vi "Set PID Params.vi"(8 "error in (no error)":errorcluster, 9 "Values":dbl[](array[numeric]), 11 "TimedPWMControl in":refnum<class "TimedPWMControl.lvclass">) -> (0 "error out":errorcluster, 3 "TimedPWMControl out":refnum<class "TimedPWMControl.lvclass">)   [LabVIEW 2020, in "VolatusControl.lvlib" / "TimedPWMControl.lvclass"]
uses:
  TimedPWMControl.lvclass
  TimedPWMControl.lvclass/TimedPWMControl.ctl
  lv-control/IG PID/Parameters.ctl
  lv-control/IG PID/IG PID.lvlib
  lv-control/IG PID/PID/PID.lvclass
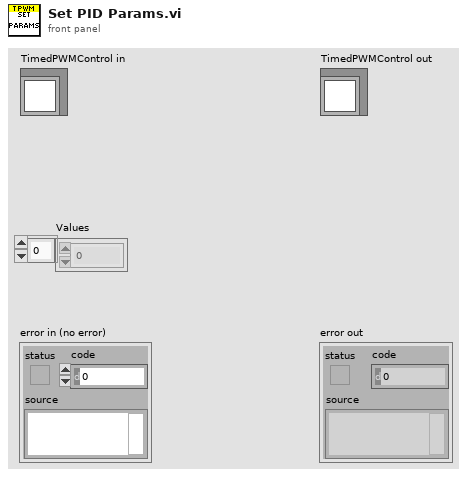
[diagram p1: front panel]
types:
  T1 = typedef "IG PID.lvlib/Parameters.ctl" = cluster{"P Band":dbl, "I Gain":dbl, "D Gain":dbl, "F Gain":dbl}
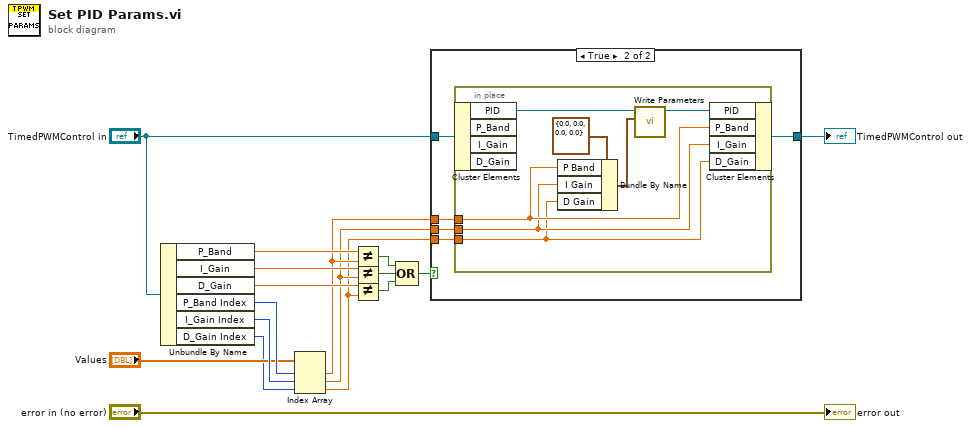
[diagram p0: block diagram]
diagram:
  n1 = Unbundle By Name("TimedPWMControl in") -> ("P_Band"=w13:dbl, "I_Gain"=w14:dbl, "D_Gain"=w12:dbl, "P_Band Index"=w15:i32, "I_Gain Index"=w16:i32, "D_Gain Index"=w2:i32)
  n2 = Index Array(array="Values", index #1=w15, index #2=w16, index #3=w2) -> (element #1=w8:dbl, element #2=w7:dbl, element #3=w3:dbl)
  n3 = Not Equal?(x=w13, y=w8) -> (x != y?=w11:bool)
  n4 = Not Equal?(x=w14, y=w7) -> (x != y?=w10:bool)
  n5 = Not Equal?(x=w12, y=w3) -> (x != y?=w9:bool)
  n6 = Compound Arithmetic op=OR(w11, w10, w9) -> (w1:bool)
  n7 = case shown="True" w1 {
    tunnel: w8 -> [_ w23]
    tunnel: w7 -> [_ w22]
    tunnel: [w18 w21] -> w6
    tunnel: "TimedPWMControl in" -> [w18 w20]
    tunnel: w3 -> [_ w19]
    frame False {
    }
    frame True {
      n8 = in-place {
        in-place-border: w23 -> [w29]
        in-place-border: w22 -> [w28]
        in-place-border: w19 -> [w27]
        n9 = in-place-cluster #1(w20) -> ("PID"=w30:refnum<class "PID.lvclass">)  [unwired: 3 out]
        n10 = Bundle By Name(cluster=T1 {"P Band"=0.0, "I Gain"=0.0, "D Gain"=0.0, "F Gain"=0.0} ("Parameters"), "P Band"=w29, "I Gain"=w28, "D Gain"=w27) -> (w25:T1)
        n11 = call "Write Parameters.vi"("Parameters"=w25, "PID in"=w30) -> ("PID out"=w24:refnum<class "PID.lvclass">)  [unwired: 8 in, 1 out]
        n12 = in-place-cluster #1("PID"=w24, "P_Band"=w29, "I_Gain"=w28, "D_Gain"=w27) -> (w21:refnum<class "TimedPWMControl.lvclass">)
      }
    }
  }
  "TimedPWMControl out" <- w6
  "error out" <- "error in (no error)"
